vi "Read_field.vi"() -> ()   [LabVIEW 2015]
uses:
  Mercury_IPS/Public/Controls/Comms Transport Layer.ctl
  Mercury_IPS/Public/Libraries/Magnet/Controls/Identifier.ctl
  Mercury_IPS/Public/Libraries/System/Open/Open System.vi
  Mercury_IPS/Public/Libraries/Magnet/Open/Open Magnet Device.vi
  Mercury_IPS/Public/Libraries/Magnet/Configuration/Read/Current to Field Factor (Read).vi
  Mercury_IPS/Public/Libraries/Magnet/Signals/Read/Current (Read).vi
  Mercury_IPS/Mercury iXX.lvlib
  Mercury_IPS/Public/Libraries/System.lvlib
  Mercury_IPS/Public/Libraries/Magnet.lvlib
panel:
  out "Magnetic Field (T)":dbl
  out "Current":dbl
  out "AtoB":dbl caption="Current Field Factor (A/T)" format="%#.1f"
  in  "Device Identifier":T1="GRPZ"
  out "error out":errorcluster
  in  "Connection Details":cluster{"Comms Layer":T2, "IP Address":string}
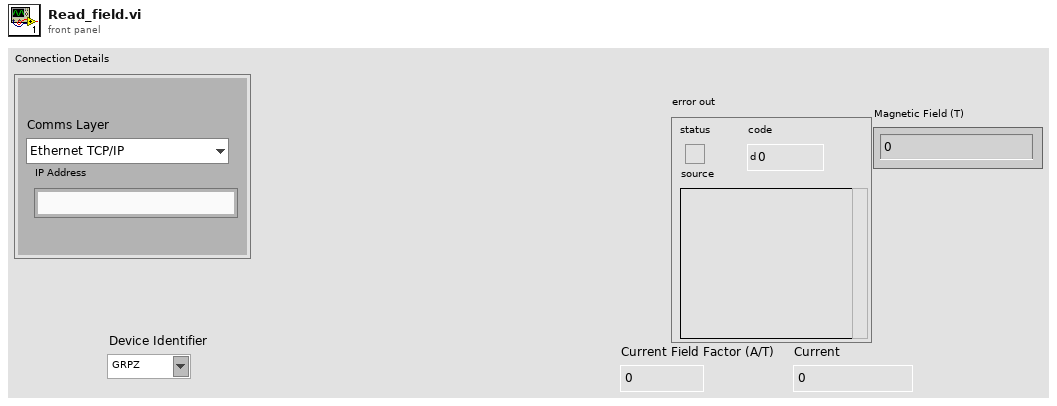
[diagram p1: front panel]
types:
  T1 = typedef "Mercury iXX.lvlib/Magnet.lvlib/Identifier.ctl" = string
  T2 = typedef "Mercury iXX.lvlib/Comms Transport Layer.ctl" = enum16{"Ethernet TCP/IP", "USB", "ISOBus - RS-232", "GPIB"}
  T3 = typedef "Mercury iXX.lvlib/Mercury Reference.ctl" = cluster{"Comms":refnum<visa-resource-name>, "Device ID":string[], "Comms Layer":T2, "Command":string, "Query reference":T4}
  T4 = typedef "Mercury iXX.lvlib/Query Dynamic Reference.ctl" = refnum<vi>
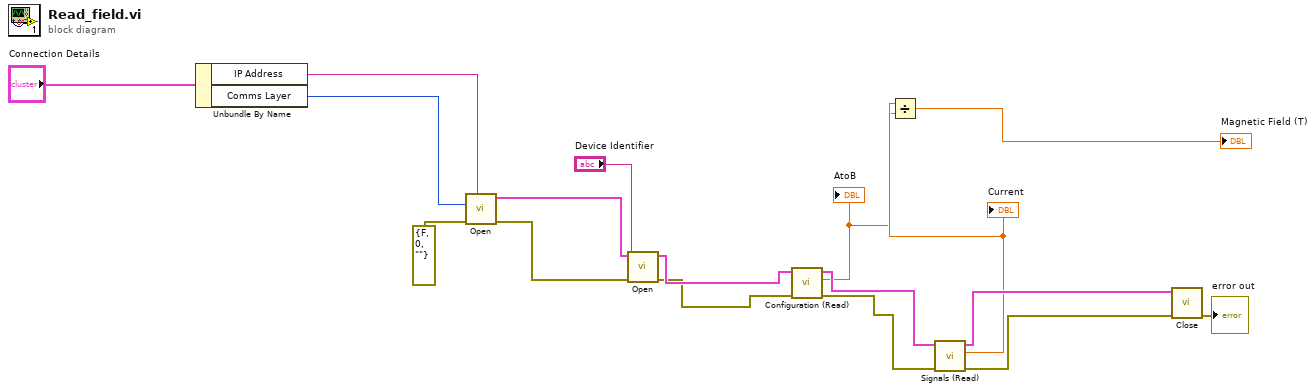
[diagram p0: block diagram]
diagram:
  n1 = Unbundle By Name("Connection Details") -> ("IP Address"=w15:string, "Comms Layer"=w14:T2)
  n2 = call-poly "Open.vi"("IP Address"=w15, "error in (no error)"=errorcluster {"status"=FALSE, "code"=0, "source"=""}, "Comms Layer"=w14) -> ("error out"=w12:errorcluster, "Mercury Reference Out"=w11:T3)  [unwired: 4 in, 3 out]
  n3 = call-poly "Open.vi"("error in (no error)"=w12, "Device Identifier"="Device Identifier", "Mercury Reference In"=w11) -> ("error out"=w8:errorcluster, "Mercury Reference Out"=w9:T3)  [unwired: 7 out]
  n4 = call-poly "Configuration (Read).vi"("error in"=w8, "Mercury Reference In"=w9) -> ("error out"=w6:errorcluster, "AtoB"=w2:dbl, "Mercury Reference Out"=w7:T3)  [unwired: 1 in, 6 out]
  "AtoB" <- w2
  n5 = call-poly "Signals (Read).vi"("error in"=w6, "Mercury Reference In"=w7) -> ("error out"=w5:errorcluster, "Current"=w3:dbl, "Mercury Reference Out"=w4:T3)  [unwired: 1 in, 6 out]
  "Current" <- w3
  n6 = Divide(x=w3, y=w2) -> (x/y=→"Magnetic Field (T)":dbl)
  n7 = call "Close.vi"("error in (no error)"=w5, "Mercury Reference"=w4) -> ("error out"=→"error out":errorcluster)  [unwired: 9 out]
